vi "_builtins_visible_label.vi"(8 "error in (no error)":errorcluster, 10 "label":enum8{"hide", "show"}(ring), 11 "GObject in":refnum<vi>) -> (0 "error out":errorcluster, 1 "was label visible?":enum8{"hide", "show"}(ring), 2 "has label?":bool, 3 "GObject out":refnum<vi>)   [LabVIEW 2019, in "Script.lvlib"]
doc: "Shows or hides the GObject label if exists.\n\nCreated by: Ryan Pacini"
uses:
  Script.lvlib
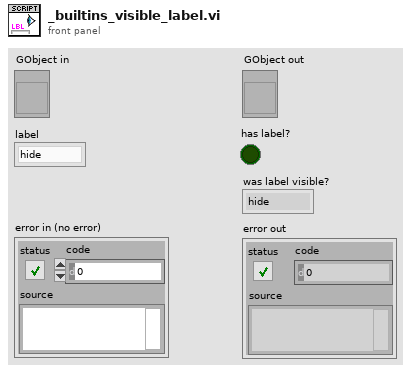
[diagram p1: front panel]
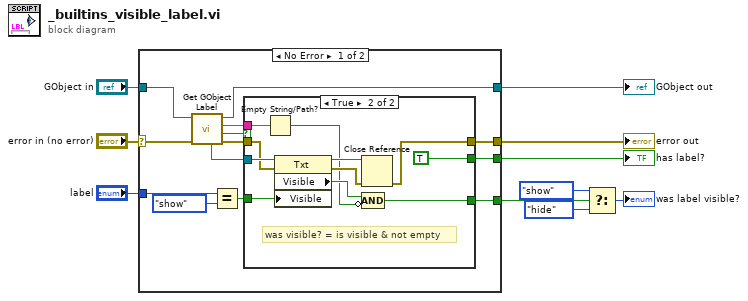
[diagram p0: block diagram]
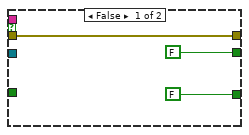
[diagram p2: hidden frame]
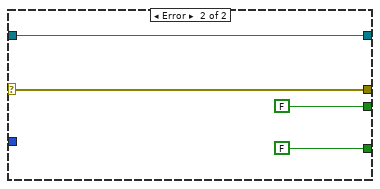
[diagram p3: hidden frame]
diagram:
  n1 = case shown="No Error" "error in (no error)" {
    selector: "error in (no error)" -> [w23 w40]
    tunnel: "label" -> [w14 _]
    tunnel: [w20 FALSE ("Visible")] -> w5
    tunnel: [w19 w40] -> w4
    tunnel: "GObject in" -> [w17 w41]
    tunnel: [w16 w41] -> w2
    tunnel: [w15 FALSE] -> w1
    frame No Error {
      n2 = call <vilib>:"Get GObject Label.vi"("error in (no error)"=w23, "GObject"=w17) -> ("error out"=w21:errorcluster, "Object Has Label?"=w18:bool, "Object Label"=w11:string, "dup GObject"=w16:refnum<vi>, "Label Reference"=w22:refnum<vi>)  [unwired: 5 in]
      n3 = Equal?(x=w14, y=enum8{"hide", "show"}."show") -> (x = y?=w13:bool)
      n4 = case shown="True" w18 {
        tunnel: w22 -> [_ w37]
        tunnel: w21 -> [w26 w36]
        tunnel: w13 -> [_ w35]
        tunnel: [FALSE ("Visible") w28] -> w20
        tunnel: [w26 w32] -> w19
        tunnel: [FALSE TRUE] -> w15
        tunnel: w11 -> [_ w30]
        frame False {
        }
        frame True {
          # "was visible? = is visible & not empty"
          n5 = Empty String/Path?(string/path=w30) -> (empty?=w27:bool)
          n6 = property class="Txt"(reference=w37, error in=w36, "Visible"=w35) -> (reference out=w34:refnum<vi>, error out=w33:errorcluster, "Visible"=w29:bool)
          n7 = Close Reference(reference=w34, error in (no error)=w33) -> (error out=w32:errorcluster)
          n8 = Compound Arithmetic op=AND(w29, invert w27) -> (w28:bool)
        }
      }
    }
    frame Error {
    }
  }
  "error out" <- w4
  "GObject out" <- w2
  "has label?" <- w1
  n9 = Select(t=enum8{"hide", "show"}."show" ("was inc/dec visible?"), s=w5, f=enum8{"hide", "show"}."hide" ("was inc/dec visible?")) -> (s? t:f=→"was label visible?":enum8{"hide", "show"})
